vi "Dynamic Load DAQmx.vi"(8 "Error In":errorcluster) -> (0 "Error Out":errorcluster, 2 "Device names":string[](array[string]), 3 "Digitizers out":refnum<class "Pulse Driver.lvclass">[](array[class]))   [LabVIEW 2016]
uses:
  Instruments/Pulse Driver/Pulse Driver.lvclass
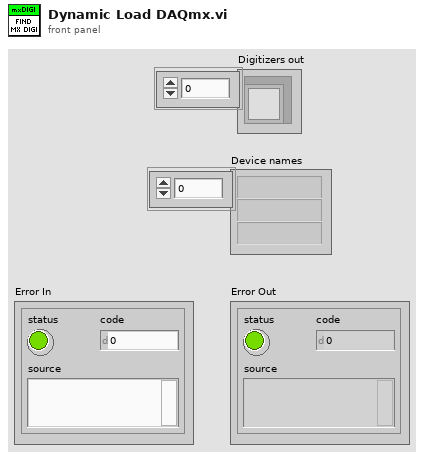
[diagram p1: front panel]
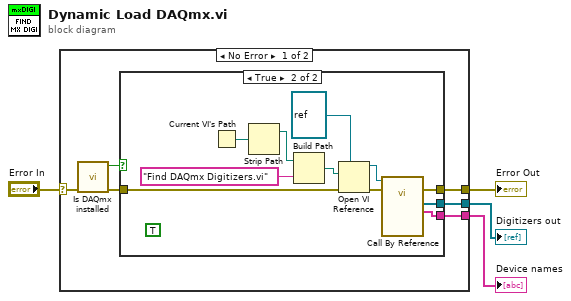
[diagram p0: block diagram]
diagram:
  n1 = case shown="No Error" "Error In" {
    selector: "Error In" -> [w8 w23]
    tunnel: [w10 w23] -> w2
    tunnel: [w6 _] -> w4
    tunnel: [w5 _] -> w3
    frame No Error {
      n2 = call "Is DAQmx installed.vi"("Error In"=w8) -> ("Error Out"=w7:errorcluster, "file or folder exists?"=w9:bool)  [unwired: 9 in]
      n3 = case shown="True" w9 {
        tunnel: w7 -> [w11 w17]
        tunnel: [w11 w14] -> w10
        tunnel: [_ w15] -> w6
        tunnel: [_ w12] -> w5
        frame False {
        }
        frame True {
          (unwired) TRUE ("DAQmx loaded")
          n4 = Current VI's Path() -> (path=w21:path)
          n5 = Strip Path(path=w21) -> (stripped path=w13:path)  [unwired: 1 out]
          n6 = Build Path(base path=w13, name or relative path="Find DAQmx Digitizers.vi") -> (appended path=w16:path)
          n7 = Open VI Reference(type specifier VI Refnum (for type only)=refnum<vi> refnum, vi path=w16, error in (no error)=w17) -> (vi reference=w19:refnum<vi>, error out=w18:errorcluster)  [unwired: 3 in]
          n8 = call-by-ref "?"(reference=w19, error in=w18) -> (error out=w14:errorcluster, "Device names"=w15:string[], "Drivers out"=w12:refnum<class "Pulse Driver.lvclass">[])  [unwired: 9 in, 2 out]
        }
      }
    }
    frame Error {
    }
  }
  "Error Out" <- w2
  "Digitizers out" <- w3
  "Device names" <- w4
